vi "www template global keys.vi"(6 "Current User":T1, 7 "ENV":T2, 8 "error in (no error)":errorcluster, 10 "Connection Refnum":T3, 11 "Template Keys In (empty)":T2) -> (0 "error out":errorcluster, 2 "Connection Refnum":T3, 3 "new Template Keys":T2)   [LabVIEW 2011]
uses:
  ITK EXT/utils/keyedarr.llb/Keyed Array.ctl
  Summitek EXT/ODBC/SQL Controls/Connection Refnum.ctl
  server/database/Users/User Record.ctl
  server/server lib/Spartan Version.vi
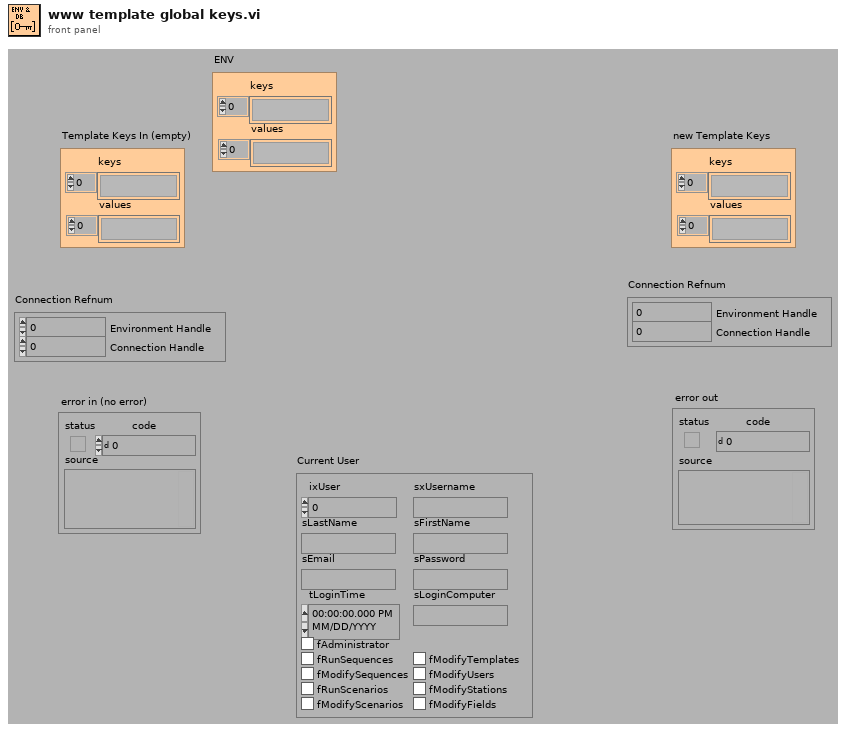
[diagram p1: front panel]
types:
  T1 = typedef "User Record.ctl" = cluster{"ixUser":i32, "sxUsername":string, "sLastName":string, "sFirstName":string, "sEmail":string, "sPassword":string, "tLoginTime":timestamp, "sLoginComputer":string, "fAdministrator":bool, "fRunSequences":bool, "fModifySequences":bool, "fRunScenarios":bool, "fModifyScenarios":bool, "fModifyTemplates":bool, "fModifyUsers":bool, "fModifyStations":bool, "fModifyFields":bool}
  T2 = typedef "Keyed Array.ctl" = cluster{"keys":string[], "values":string[]}
  T3 = typedef "Connection Refnum.ctl" = cluster{"Environment Handle":i32, "Connection Handle":i32}
  T4 = typedef "OGAB Version.ctl" = cluster{"Version":string, "Build Number":u32, "Build Date/Time":dbl}
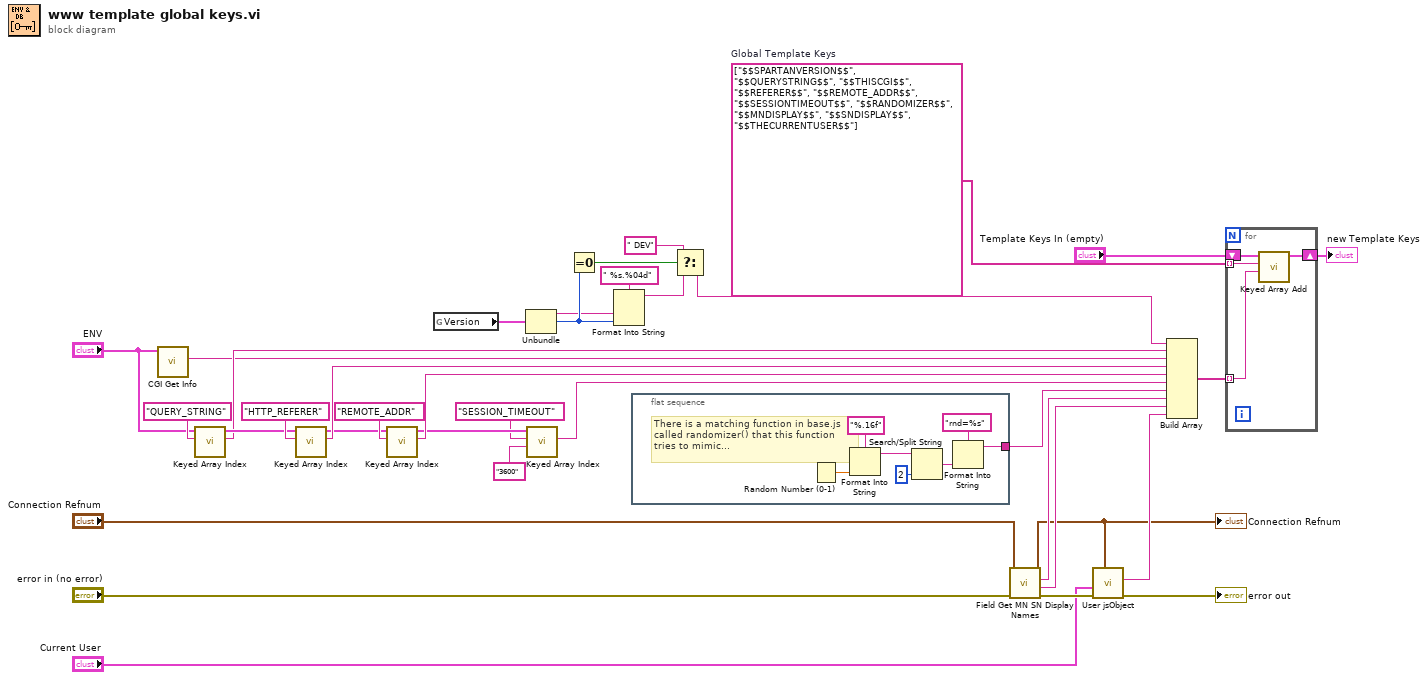
[diagram p0: block diagram]
diagram:
  w30 = string[] ["$$SPARTANVERSION$$", "$$QUERYSTRING$$", "$$THISCGI$$", "$$REFERER$$", "$$REMOTE_ADDR$$", "$$SESSIONTIMEOUT$$", "$$RANDOMIZER$$", "$$MNDISPLAY$$", "$$SNDISPLAY$$", "$$THECURRENTUSER$$"]  # Global Template Keys
  n1 = call "CGI Get Info.vi"("env"="ENV") -> ("virtual path"=w28:string)  [unwired: 6 out]
  n2 = call "Keyed Array Index.vi"("key"="QUERY_STRING" ("name"), "array in"="ENV") -> ("value"=w29:string, "duplicate array"=w33:T2)  [unwired: 2 in, 2 out]
  n3 = call "Keyed Array Index.vi"("key"="HTTP_REFERER", "array in"=w33) -> ("value"=w27:string, "duplicate array"=w20:T2)  [unwired: 2 in, 2 out]
  n4 = call "Keyed Array Index.vi"("key"="REMOTE_ADDR", "array in"=w20) -> ("value"=w19:string, "duplicate array"=w5:T2)  [unwired: 2 in, 2 out]
  n5 = global read "Spartan Version.vi" "Version"() -> (w18:T4)
  n6 = Unbundle(w18) -> ("Version"=w9:string, "Build Number"=w14:u32)  [unwired: 1 out]
  n7 = call "Keyed Array Index.vi"("default value"="3600", "key"="SESSION_TIMEOUT", "array in"=w5) -> ("value"=w2:string)  [unwired: 1 in, 3 out]
  n8 = Equal To 0?(x=w14) -> (x = 0?=w10:bool)
  n9 = Format Into String(format string=" %s.%04d", w9, w14) -> (resulting string=w11:string)  [unwired: 2 in, 1 out]
  n10 = flat-sequence {
    tunnel: [w37] -> w7
    frame #0 {
      # "There is a matching function in base.js\ncalled randomizer() that this function\ntries to mimic..."
      n11 = Random Number (0-1)() -> (number: 0 to 1=w43:dbl)
      n12 = Format Into String(format string="%.16f", w43) -> (resulting string=w38:string)  [unwired: 2 in, 1 out]
      n13 = Search/Split String(string=w38, offset (0)=2) -> (match + rest of string=w40:string)  [unwired: 3 out]
      n14 = Format Into String(format string="rnd=%s", w40) -> (resulting string=w37:string)  [unwired: 2 in, 1 out]
    }
  }
  n15 = Select(t=" DEV", s=w10, f=w11) -> (s? t:f=w12:string)
  n16 = call "Field Get MN SN Display Names.vi"("error in (no error)"="error in (no error)", "Connection Refnum"="Connection Refnum") -> ("error out"=w17:errorcluster, "Serial Number Display Name"=w25:string, "Model Number Display Name"=w26:string, "Connection Refnum"=w1:T3)  [unwired: 6 out]
  "Connection Refnum" <- w1
  n17 = call "User jsObject.vi"("DB Connection Ref"=w1, "error in (no error)"=w17, "User Record (empty)"="Current User") -> ("error out"=→"error out":errorcluster, "User Literal Object"=w6:string)  [unwired: 2 in, 5 out]
  n18 = Build Array(w12, w29, w28, w27, w19, w2, w7, w26, w25, w6) -> (w24:string[])
  n19 = for {
    shift-right: [w46] -> w22
    shift-left: "Template Keys In (empty)" -> [w47]
    tunnel: w30 -> [w45] mode=indexing
    tunnel: w24 -> [w44] mode=indexing
    n20 = call "Keyed Array Add.vi"("value"=w44, "key"=w45, "array in"=w47) -> ("array out"=w46:T2)  [unwired: 1 in, 3 out]
  }
  "new Template Keys" <- w22
